vi "Auto Shooter Mode.vi"(0 "Shooter Command":T1, 9 "Ball Loaded?":bool) -> (8 "Secure Ball?":bool, 10 "Angle In Range?":bool, 11 "RPM Ready?":bool, 12 "Vision Target Aligned?":bool, 13 "Intake High Angle Allowed?":bool, 14 "State":T5, 15 "Shooter Ready?":bool, 16 "Left Output":dbl, 17 "Right Output":dbl, 18 "Angle Motor Output":dbl, 19 "Trigger Output":dbl)   [LabVIEW 2015]
uses:
  Common Code/Shooter State.ctl
  Common Code/Shooter Command Cluster.ctl
  Common Code/Shooter Commands.ctl
  Common Code/Shoot Modes Enum.ctl
  Common Code/Shot Type.ctl
  Common Code/Change Detect Int.vi
  Common Code/Change Detect Boolean.vi
  Robot Global Data.vi
panel:
  out "Ball Loaded? 2":bool
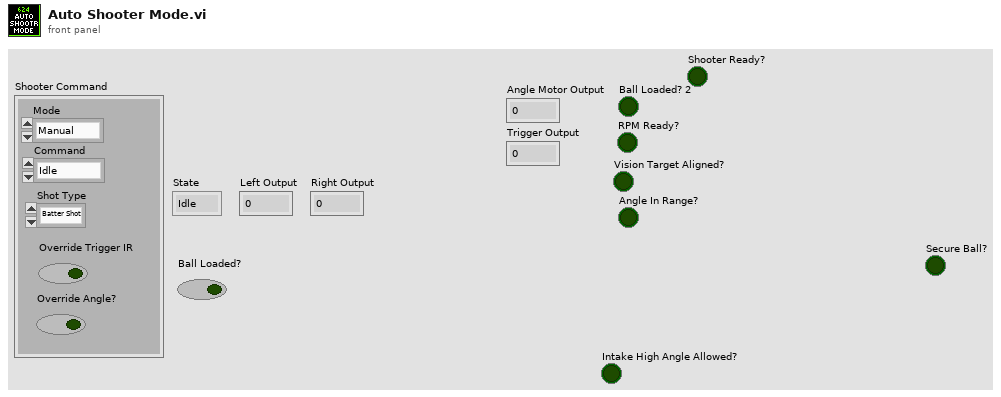
[diagram p1: front panel]
types:
  T1 = typedef "Shooter Command Cluster.ctl" = cluster{"Command":T2, "Mode":T3, "Shot Type":T4, "Override Trigger IR":bool, "Override Angle?":bool}
  T2 = typedef "Shooter Commands.ctl" = enum16{"Idle", "Prime Shooter", "Shoot"}
  T3 = typedef "Shoot Modes Enum.ctl" = enum16{"Manual", "Safe", "Auto"}
  T4 = typedef "Shot Type.ctl" = enum16{"Batter Shot", "Corner Shot", "Curve Shot", "Vision Shot", "Deep Middle Shot"}
  T5 = typedef "Shooter State.ctl" = enum16{"Idle", "Warmup", "Shooter Ready", "Shoot"}
  T6 = typedef "Intake Status Cluster.ctl" = cluster{"Roller Power":dbl, "Angle Power":dbl, "Intake Mode":T7, "Intake States":T8, "Rollers Active?":bool, "Current Height":dbl, "Target Height":dbl, "Encoder Raw Position":dbl, "Forward Tripped?":bool, "Backward Tripped?":bool, "Override IR?":bool}
  T7 = typedef "Intake Mode.ctl" = enum16{"Safe", "Auto", "Manual"}
  T8 = typedef "Intake States.ctl" = enum16{"Idle", "Set roller speed", "Move to angle"}
  T9 = typedef "Drivetrain Status Cluster.ctl" = cluster{"Modes":T10, "Y (Throttle)":dbl, "X (Steer)":dbl, "Gyro In Range?":bool, "Distance Drive Finished?":bool, "Stop Eject Lockout":bool, "Dist Drive Status":T11, "Y Target":dbl, "Heading Target":dbl, "Vision Target Aligned?":bool, "Gear":dbl, "1st Gear Time":dbl, "2nd Gear Time":dbl, "1st Gear Shifts":dbl, "2nd Gear Shifts":dbl}
  T10 = typedef "Drivetrain Modes.ctl" = enum16{"Climb", "Manual", "Ball Vision Targeting", "Goal Vision Targeting", "PID Distance Drive", "Hybrid"}
  T11 = typedef "Dist Drive Status.ctl" = cluster{"Y In Range":bool, "X In Range":bool, "Gyro In Range":bool, "Y Dist":dbl, "X Dist":dbl, "Gyro":dbl}
  T12 = typedef "Dashboard Control Data.ctl" = cluster{"Shooter Presets":T13, "Encoder Control":T15, "Steer PID output":cluster{"output high":dbl, "output low":dbl}, " Steer PID gains":cluster{"proportional gain (Kc)":dbl, "integral time (Ti, min)":dbl, "derivative time (Td, min)":dbl}, "Drivetrain Settings":T16, "Vision Packet":T17, "Dashboard Drivetrain Command":T18, "Info/Command Cluster":T20, "Ball Vision Packet":T21, "Intake Presets":T23, "Intake Encoder Control":T25, "Climb Presets":T26, "Ultrasonic Limit":dbl, "Roll Limit":dbl, "Pitch Limit":dbl, "Goal Output Range":cluster{"output high":dbl, "output low":dbl}}
  T13 = typedef "Shooter Presets.ctl" = cluster{"Batter Shot":T14, "Deep Middle Shot":T14, "Manual Shot":T14, "Left Ticks Per Rotation":dbl, "Right Ticks Per Rotation":dbl, "Low Bar Shot":T14, "Shooter RPM Tolerance":dbl, "IIR Filter Power":dbl, "Trigger Power":dbl, "Fire from Load Delay":i32, "Angle Pot M":dbl, "Angle Pot B":dbl, "Shooter Length":dbl, "String Pot Dist":dbl, "Angle PID gains":cluster{"proportional gain (Kc)":dbl, "integral time (Ti, min)":dbl, "derivative time (Td, min)":dbl}, "Angle Motor Output":cluster{"output high":dbl, "output low":dbl}, "Shooter Angle Tolerance":dbl, "Vision Shoot x^2":dbl, "Vision Shoot x":dbl, "Dist from Axis Cam to Pivot":dbl, "High Goal Center Height":dbl, "Feed Forward Max Accel":dbl, "Feed Forward Kv":dbl, "Backwards Trigger":dbl, "Shot Finish Delay (ms)":dbl, "Angle Max Current":dbl, "Angle Current Trip Time":dbl, "Shooter Intake Angle":dbl, "Vision Shoot c":dbl, "Reset?":bool, "Servo Release Delay":dbl, "Servo Idle Angle":i32, "Servo Hold Angle":i32, "Angle Pot x^2":dbl, "Angle Pot x":dbl, "Angle Pot c":dbl, "Ignore Angle?":bool}
  T14 = typedef "Shot Presets.ctl" = cluster{"Left Wheel RPM":dbl, "Right Wheel RPM":dbl, "Angle":dbl}
  T15 = typedef "Encoder Control.ctl" = cluster{"Right Tick Constant":dbl, "Left Tick Constant":dbl, "Reset?":bool, "Y Dist":cluster{"PID gains":cluster{"proportional gain (Kc)":dbl, "integral time (Ti, min)":dbl, "derivative time (Td, min)":dbl}}, "Y Stop Thresh":dbl, "Y Stop Speed":dbl}
  T16 = typedef "Drivetrain Settings.ctl" = cluster{"Gyro Tolerance":dbl, "Throttle Ramp (ms)":dbl, "Angular rate compensation":bool, "Throttle to Rate Scale":dbl, "Rate compensation gain":dbl, "Kv":dbl, "Ka":dbl, "Feed Forward P":dbl, "Feed Forward D":dbl, "Goal Vision PID gains":cluster{"proportional gain (Kc)":dbl, "integral time (Ti, min)":dbl, "derivative time (Td, min)":dbl}, "Goal Detection Window":dbl}
  T17 = typedef "Goal Vision Packet.ctl" = cluster{"Distance":dbl, "Center X":dbl, "Center Y":dbl, "Found Target?":bool}
  T18 = typedef "Dashboard Drivetrain Command.ctl" = cluster{"Drivetrain Vision":T19}
  T19 = typedef "Drivetrain Vision.ctl" = cluster{"Goal Window":dbl, "Ball Window":dbl}
  T20 = typedef "Ball Tracking Command Cluster.ctl" = cluster{"Distance to Ball":dbl, "Desired Angle":dbl, "Command":enum16{"Turn to Ball", "Turn to Angle", "Get Distance"}, "Pixels from Center":dbl}
  T21 = typedef "Ball Vision Packet.ctl" = cluster{"Ball Detected?":bool, "Distance to Ball":dbl, "Desired Angle":dbl, "Pixels from Center":dbl, "Tracking mode":T22}
  T22 = typedef "Tracking Mode.ctl" = enum16{"Turn to Ball", "Turn to Angle"}
  T23 = typedef "Intake Presets.ctl" = cluster{"Intake Speed":dbl, "Outake Speed":dbl, "Low Height":dbl, "Half Height":dbl, "Full Height":dbl, "Angle Speed":dbl, "Fast Angle":dbl, "Encoder Scale":dbl, "Load Height":dbl, "Output Range":T24, "Rotation Power Max/Min":dbl, "MaxCurrent":dbl, "Intake Trip Time":dbl, "Idle Height":dbl, "Max Height":dbl, "Reset Encoders?":bool, "PID gains":cluster{"proportional gain (Kc)":dbl, "integral time (Ti, min)":dbl, "derivative time (Td, min)":dbl}}
  T24 = typedef "Drivetrain Output Range.ctl" = cluster{"output high":dbl, "output low":dbl}
  T25 = typedef "IntakeEcoderControl.ctl" = cluster{"Arm Tick Constant":dbl, "Reset?":bool, "Y Dist":cluster{"PID gains":cluster{"proportional gain (Kc)":dbl, "integral time (Ti, min)":dbl, "derivative time (Td, min)":dbl}}, "Y Stop Thresh":dbl, "Y Stop Speed":dbl}
  T26 = typedef "Climb Presets.ctl" = cluster{"Pull Power":dbl, "Unpin Power":dbl, "Time to Hold":dbl}
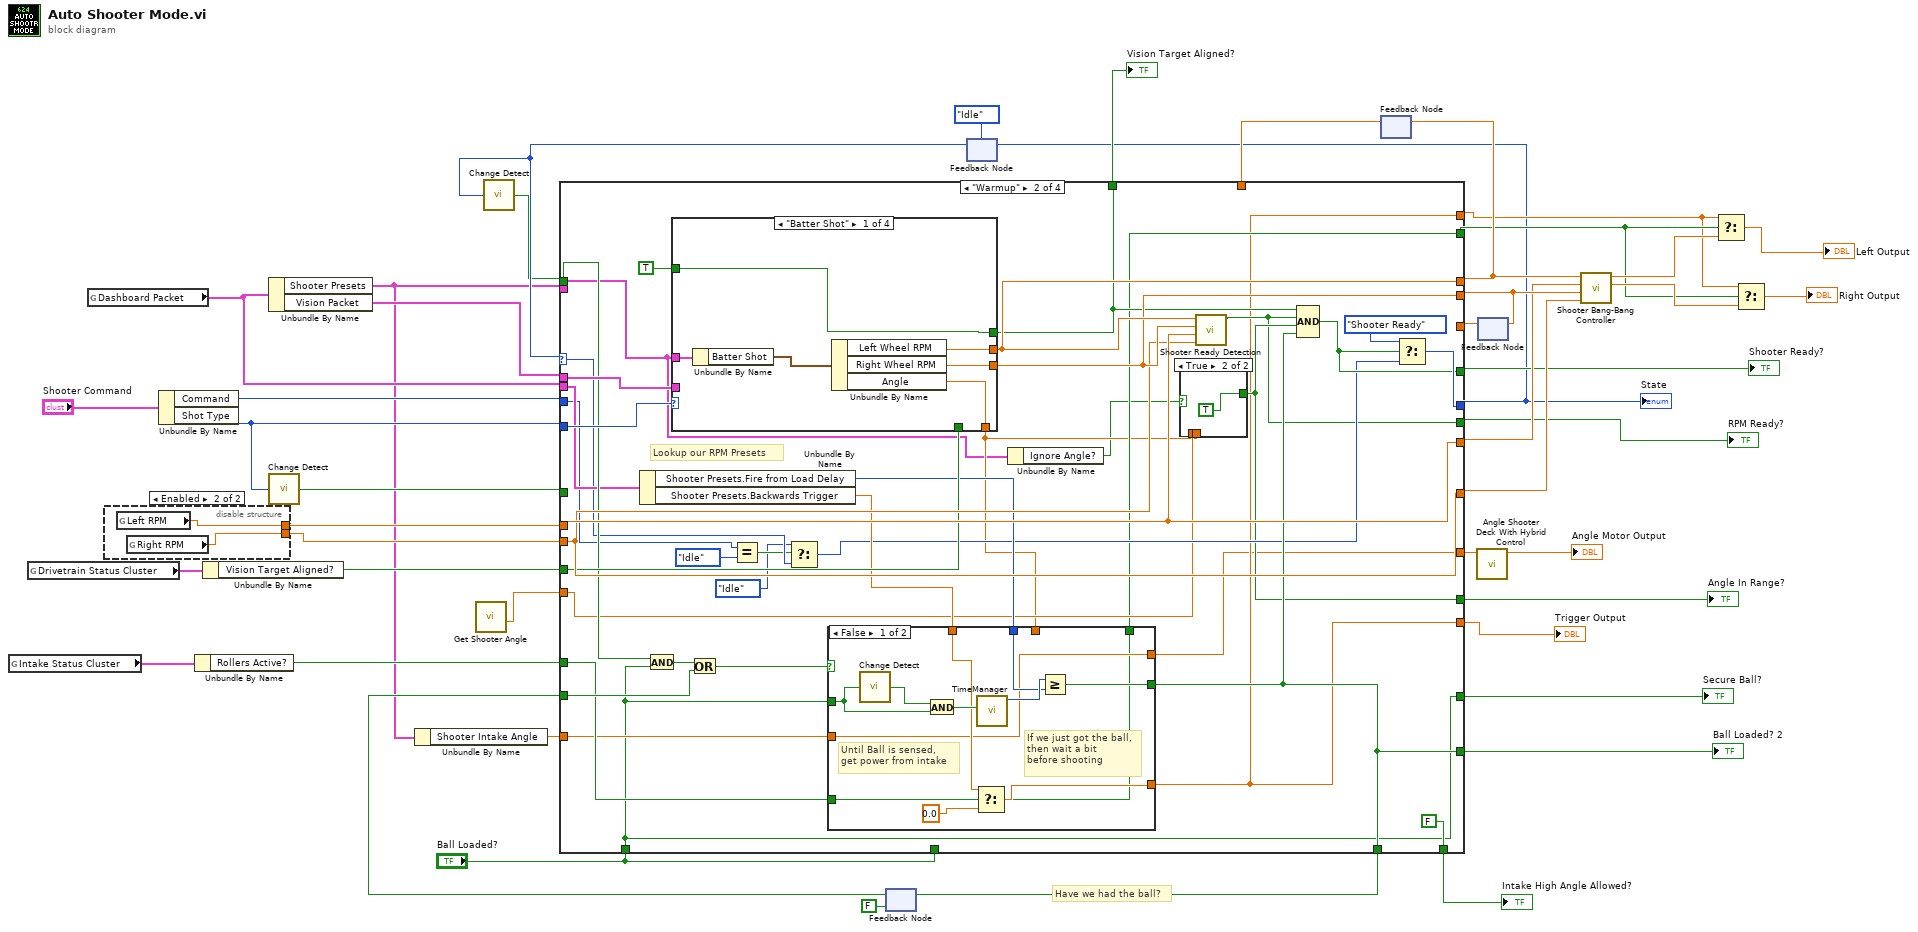
[diagram p0: block diagram]
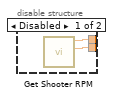
[diagram p2: hidden frame]
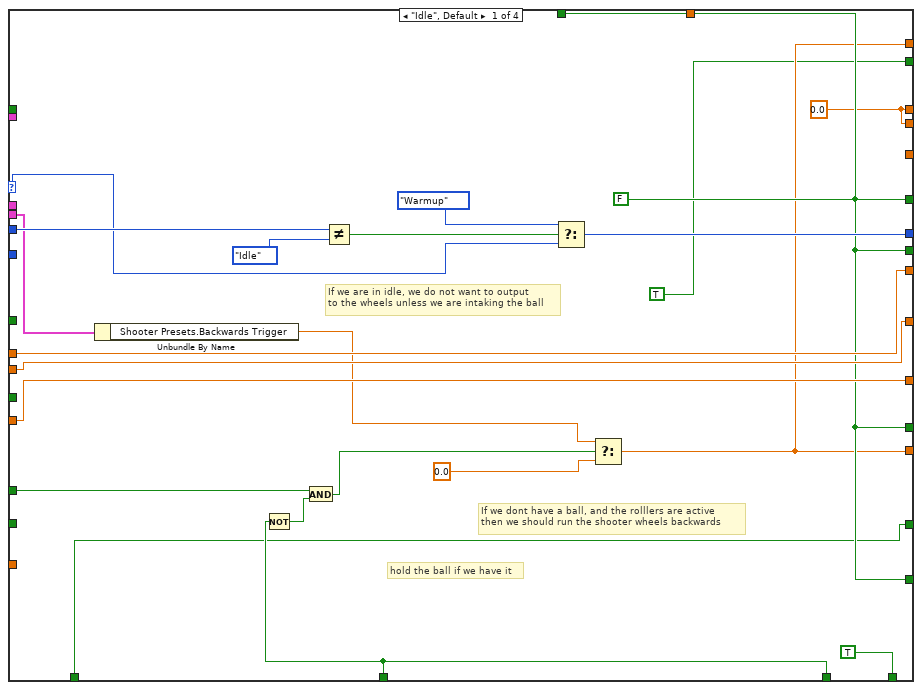
[diagram p3: hidden frame]
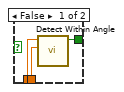
[diagram p4: hidden frame]
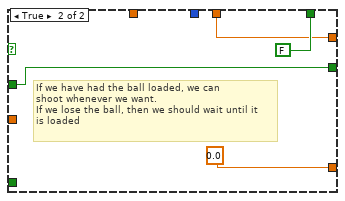
[diagram p5: hidden frame]
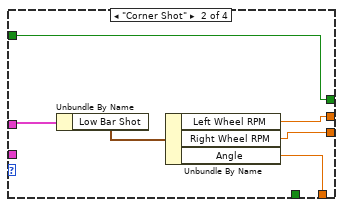
[diagram p6: hidden frame]
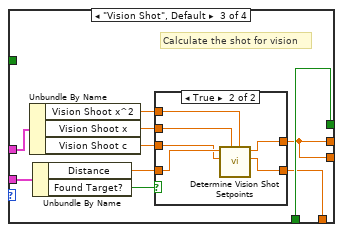
[diagram p7: hidden frame]
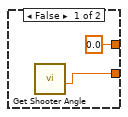
[diagram p8: hidden frame]
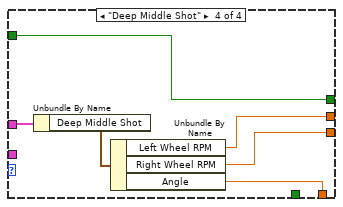
[diagram p9: hidden frame]
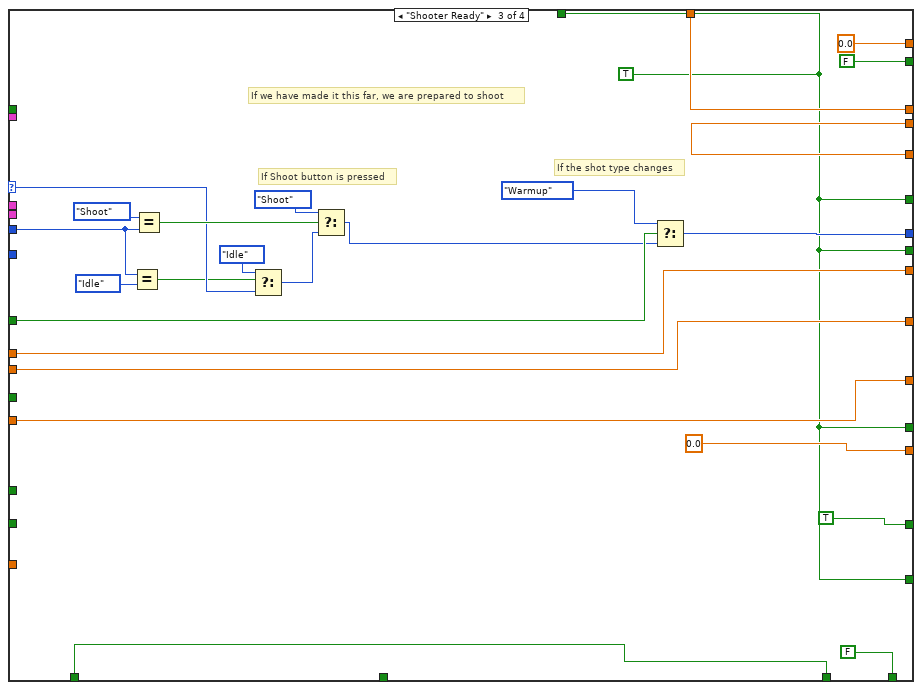
[diagram p10: hidden frame]
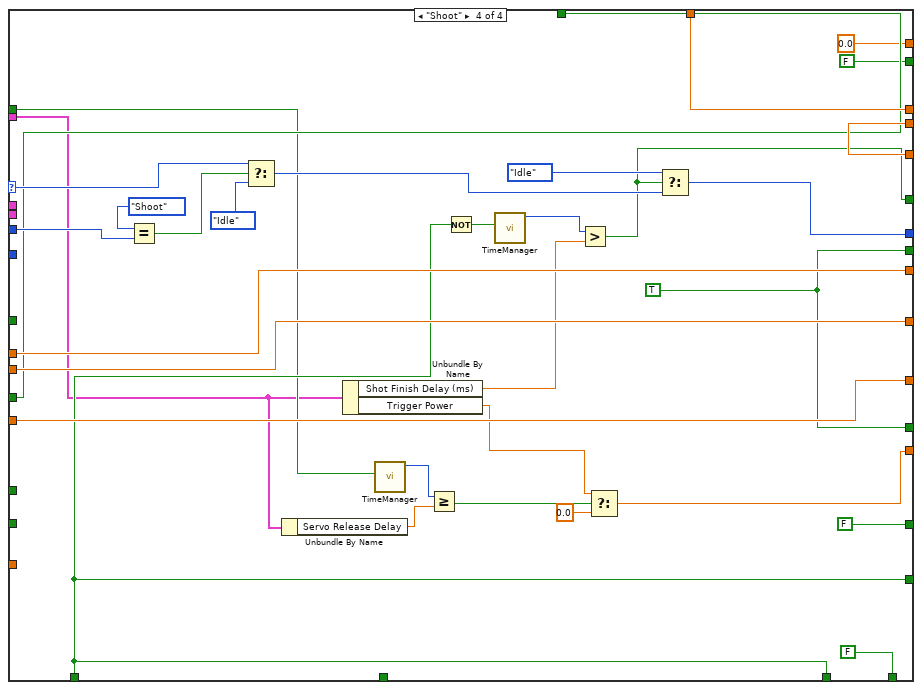
[diagram p11: hidden frame]
diagram:
  # "Have we had the ball?"
  n1 = global read "Robot Global Data.vi" "Intake Status Cluster"() -> (w5:T6)
  n2 = global read "Robot Global Data.vi" "Drivetrain Status Cluster"() -> (w32:T9)
  n3 = global read "Robot Global Data.vi" "Dashboard Packet"() -> (w7:T12)
  n4 = disable-structure shown="Enabled" {
    disable-tunnel: [w47 w48] -> w36
    disable-tunnel: [w46 w49] -> w35
    frame Disabled {
      n5 = call "Get Shooter RPM.vi"() -> ("Right RPM"=w46:dbl, "Left RPM"=w47:dbl)  [unwired: 9 in, 1 out]
    }
    frame Enabled {
      n6 = global read "Robot Global Data.vi" "Left RPM"() -> (w48:dbl)
      n7 = global read "Robot Global Data.vi" "Right RPM"() -> (w49:dbl)
    }
  }
  n8 = Unbundle By Name("Shooter Command") -> ("Command"=w44:T2, "Shot Type"=w42:T4)
  n9 = Unbundle By Name(w5) -> ("Rollers Active?"=w30:bool)
  n10 = Unbundle By Name(w32) -> ("Vision Target Aligned?"=w31:bool)
  n11 = Unbundle By Name(w7) -> ("Shooter Presets"=w6:T13, "Vision Packet"=w20:T17)
  n12 = call-poly "Change Detect.vi"("In"=w42) -> ("Changed?"=w41:bool)
  n13 = Unbundle By Name(w6) -> ("Shooter Intake Angle"=w4:dbl)
  n14 = call "Get Shooter Angle.vi"() -> ("Current Angle"=w8:dbl)  [unwired: 11 in]
  n15 = feedback #1(FALSE ("Ball Loaded?")) -> (w26:bool)
  n16 = feedback #2(Shooter_State."Idle") -> (w24:T5)
  n17 = call-poly "Change Detect.vi"("In"=w24) -> ("Changed?"=w23:bool)
  n18 = feedback #3() -> (w39:dbl)  [unwired: 1 in]
  n19 = feedback #4() -> (w37:dbl)  [unwired: 1 in]
  n20 = case shown="\"Warmup\"" w24 {
    selector: w24 -> [w64 w89 w174 w219]
    tunnel: w44 -> [w67 w86 w182 w222]
    tunnel: [w69 w106 w187 w212] -> w1
    tunnel: w6 -> [_ w73 _ w198]
    tunnel: w42 -> [_ w110 _ _]
    tunnel: [w55 w108 w185 w217] -> w38
    tunnel: [w55 w109 w186 w218] -> w40
    tunnel: w41 -> [_ _ w189 _]
    tunnel: w39 -> [_ _ w186 w218]
    tunnel: w37 -> [_ _ w185 w217]
    tunnel: w36 -> [w66 w105 w184 w216]
    tunnel: w35 -> [w65 w104 w183 w215]
    tunnel: [w66 w105 w184 w216] -> w34
    tunnel: [w65 w104 w183 w215] -> w33
    tunnel: w31 -> [_ w100 _ w208]
    tunnel: "Ball Loaded?" -> [w61 _ _ _]
    tunnel: w20 -> [_ w103 _ _]
    tunnel: [w62 w77 w176 w211] -> w21
    tunnel: w30 -> [w60 w93 _ _]
    tunnel: [w53 w79 0.0 ("f") w192] -> w29
    tunnel: "Ball Loaded?" -> [w50 w74 w181 w202]
    tunnel: w7 -> [w58 w90 _ _]
    tunnel: [w61 w98 w181 w202] -> w27
    tunnel: w26 -> [_ w95 _ _]
    tunnel: w23 -> [_ w94 _ w199]
    tunnel: w8 -> [w62 w82 w176 w211]
    tunnel: [w57 w102 w170 w201] -> w19
    tunnel: [w57 w83 w170 w209] -> w18
    tunnel: [w57 w81 w170 w209] -> w17
    tunnel: [w57 w98 w170 w202] -> w16
    tunnel: [w57 w101 w170 w208] -> w15
    tunnel: [TRUE w80 FALSE FALSE] -> w12
    tunnel: [w53 w79 0.0 ("f") 0.0 ("f")] -> w11
    tunnel: w4 -> [_ w76 _ _]
    tunnel: [TRUE ("Intake High Angle Allowed?") FALSE ("Intake High Angle Allowed?") FALSE ("Intake High Angle Allowed?") FALSE ("Intake High Angle Allowed?")] -> w3
    tunnel: [w50 w74 TRUE ("Intake High Angle Allowed?") FALSE ("Intake High Angle Allowed?")] -> w2
    frame "Idle", Default {
      w55 = 0.0 ("Left Wheel RPM")
      w57 = FALSE ("Shooter Ready?")
      # "hold the ball if we have it"
      # "If we dont have a ball, and the rolllers are active\nthen we should run the shooter wheels backwards"
      # "If we are in idle, we do not want to output\nto the wheels unless we are intaking the ball"
      n21 = Unbundle By Name(w58) -> ("Shooter Presets.Backwards Trigger"=w56:dbl)
      n22 = Not(x=w61) -> (.not. x?=w59:bool)
      n23 = And(x=w60, y=w59) -> (x .and. y?=w54:bool)
      n24 = Not Equal?(x=w67, y=Shooter_Commands."Idle" ("Command")) -> (x != y?=w70:bool)
      n25 = Select(t=Shooter_State."Warmup", s=w70, f=w64) -> (s? t:f=w69:T5)
      n26 = Select(t=w56, s=w54, f=0.0) -> (s? t:f=w53:dbl)
    }
    frame "Warmup" {
      # "Lookup our RPM Presets"
      n27 = Unbundle By Name(w90) -> ("Shooter Presets.Fire from Load Delay"=w92:i32, "Shooter Presets.Backwards Trigger"=w91:dbl)
      n28 = And(x=w94, y=w74) -> (x .and. y?=w96:bool)
      n29 = case shown="\"Batter Shot\"" w110 {
        tunnel: w73 -> [w135 w141 w150 w165]
        tunnel: [w133 w137 w145 w163] -> w109
        tunnel: [w132 w138 w145 w162] -> w108
        tunnel: w103 -> [_ _ w147 _]
        tunnel: [w131 w136 w151 w161] -> w101
        tunnel: w100 -> [_ _ w151 _]
        tunnel: TRUE -> [w131 w136 _ w161]
        tunnel: [w130 w139 w146 w160] -> w78
        frame "Batter Shot" {
          n30 = Unbundle By Name(w135) -> ("Batter Shot"=w134:T14)
          n31 = Unbundle By Name(w134) -> ("Left Wheel RPM"=w133:dbl, "Right Wheel RPM"=w132:dbl, "Angle"=w130:dbl)
        }
        frame "Corner Shot" {
          n32 = Unbundle By Name(w141) -> ("Low Bar Shot"=w140:T14)
          n33 = Unbundle By Name(w140) -> ("Left Wheel RPM"=w137:dbl, "Right Wheel RPM"=w138:dbl, "Angle"=w139:dbl)
        }
        frame "Vision Shot", Default {
          # "Calculate the shot for vision"
          n34 = Unbundle By Name(w150) -> ("Vision Shoot x^2"=w143:dbl, "Vision Shoot x"=w144:dbl, "Vision Shoot c"=w142:dbl)
          n35 = Unbundle By Name(w147) -> ("Distance"=w149:dbl, "Found Target?"=w148:bool)
          n36 = case shown="True" w148 {
            tunnel: w149 -> [_ w159]
            tunnel: [w152 w158] -> w146
            tunnel: [0.0 ("Power") w157] -> w145
            tunnel: w144 -> [_ w156]
            tunnel: w143 -> [_ w155]
            tunnel: w142 -> [_ w154]
            frame False {
              n37 = call "Get Shooter Angle.vi"() -> ("Current Angle"=w152:dbl)  [unwired: 11 in]
            }
            frame True {
              n38 = call "Determine Vision Shot Setpoints.vi"("x^2"=w155, "x"=w156, "c"=w154, "Distance from Target"=w159) -> ("Angle"=w158:dbl, "RPM Power"=w157:dbl)  [unwired: 6 in]
            }
          }
        }
        frame "Deep Middle Shot" {
          n39 = Unbundle By Name(w165) -> ("Deep Middle Shot"=w164:T14)
          n40 = Unbundle By Name(w164) -> ("Left Wheel RPM"=w163:dbl, "Right Wheel RPM"=w162:dbl, "Angle"=w160:dbl)
        }
      }
      n41 = Or(x=w96, y=w95) -> (x .or. y?=w97:bool)
      n42 = Equal?(x=w86, y=Shooter_Commands."Idle") -> (x = y?=w87:bool)
      n43 = Select(t=Shooter_State."Idle", s=w87, f=w89) -> (s? t:f=w88:T5)
      n44 = case shown="False" w97 {
        tunnel: w92 -> [w122 _]
        tunnel: w74 -> [w121 w129]
        tunnel: [w120 w129] -> w98
        tunnel: [w118 0.0 ("f")] -> w79
        tunnel: w93 -> [w115 _]
        tunnel: w91 -> [w117 _]
        tunnel: [w115 FALSE] -> w80
        tunnel: w78 -> [_ w126]
        tunnel: [w116 w126] -> w77
        tunnel: w76 -> [w116 _]
        frame False {
          # "Until Ball is sensed,\nget power from intake"
          # "If we just got the ball,\nthen wait a bit\nbefore shooting"
          n45 = call-poly "Change Detect.vi"("In"=w121) -> ("Changed?"=w125:bool)
          n46 = And(x=w125, y=w121) -> (x .and. y?=w124:bool)
          n47 = Select(t=w117, s=w115, f=0.0 ("t")) -> (s? t:f=w118:dbl)
          n48 = call "TimeManager.vi"("Reset?"=w124) -> ("Time Since Reset"=w123:u32)  [unwired: 9 in, 1 out]
          n49 = Greater Or Equal?(x=w123, y=w122) -> (x >= y?=w120:bool)
        }
        frame True {
          # "If we have had the ball loaded, we can\nshoot whenever we want.\nIf we lose the ball, then we should wait until it\nis loaded"
        }
      }
      n50 = Unbundle By Name(w73) -> ("Ignore Angle?"=w72:bool)
      n51 = case shown="True" w72 {
        tunnel: [w113 TRUE ("In Range?")] -> w83
        tunnel: w82 -> [w112 _]
        tunnel: w78 -> [w111 _]
        frame False {
          n52 = call "Detect Within Angle.vi"("Angle Target"=w111, "Current Angle"=w112) -> ("In Range?"=w113:bool)  [unwired: 9 in]
        }
        frame True {
        }
      }
      n53 = call "Shooter Ready Detection.vi"("Right RPM"=w104, "Left RPM"=w105, "Right RPM Target"=w108, "Left RPM Target"=w109) -> ("Shooter Ready?"=w81:bool)  [unwired: 7 in]
      n54 = Compound Arithmetic op=AND(w101, w81, w83, w98) -> (w102:bool)
      n55 = Select(t=Shooter_State."Shooter Ready", s=w102, f=w88) -> (s? t:f=w106:T5)
    }
    frame "Shooter Ready" {
      w170 = TRUE ("Vision Target Aligned?")
      # "If the shot type changes"
      # "If Shoot button is pressed"
      # "If we have made it this far, we are prepared to shoot"
      n56 = Equal?(x=w182, y=Shooter_Commands."Idle") -> (x = y?=w173:bool)
      n57 = Equal?(x=Shooter_Commands."Shoot", y=w182) -> (x = y?=w180:bool)
      n58 = Select(t=Shooter_State."Idle", s=w173, f=w174) -> (s? t:f=w175:T5)
      n59 = Select(t=Shooter_State."Shoot", s=w180, f=w175) -> (s? t:f=w178:T5)
      n60 = Select(t=Shooter_State."Warmup", s=w189, f=w178) -> (s? t:f=w187:T5)
    }
    frame "Shoot" {
      w209 = TRUE ("Vision Target Aligned?")
      n61 = Equal?(x=Shooter_Commands."Shoot", y=w222) -> (x = y?=w220:bool)
      n62 = Select(t=w219, s=w220, f=Shooter_State."Idle") -> (s? t:f=w213:T5)
      n63 = Unbundle By Name(w198) -> ("Servo Release Delay"=w197:dbl)
      n64 = Unbundle By Name(w198) -> ("Shot Finish Delay (ms)"=w204:dbl, "Trigger Power"=w194:dbl)
      n65 = call "TimeManager.vi"("Reset?"=w199) -> ("Time Since Reset"=w196:u32)  [unwired: 9 in, 1 out]
      n66 = Greater Or Equal?(x=w196, y=w197) -> (x >= y?=w195:bool)
      n67 = Not(x=w202) -> (.not. x?=w205:bool)
      n68 = call "TimeManager.vi"("Reset?"=w205) -> ("Time Since Reset"=w203:u32)  [unwired: 9 in, 1 out]
      n69 = Greater?(x=w203, y=w204) -> (0:w201:bool)
      n70 = Select(t=w194, s=w195, f=0.0) -> (s? t:f=w192:dbl)
      n71 = Select(t=Shooter_State."Idle" ("f"), s=w201, f=w213) -> (s? t:f=w212:T5)
    }
  }
  "State" <- w1
  "Trigger Output" <- w29
  "Ball Loaded? 2" <- w16
  "Shooter Ready?" <- w19
  "RPM Ready?" <- w17
  "Angle In Range?" <- w18
  "Vision Target Aligned?" <- w15
  "Intake High Angle Allowed?" <- w3
  "Secure Ball?" <- w2
  n72 = feedback-in #1(w27) -> ()
  n73 = feedback-in #2(w1) -> ()
  n74 = feedback-in #3(w40) -> ()
  n75 = call "Angle Shooter Deck With Hybrid Control.vi"("Target Angle"=w21) -> ("Angle Motor Power Out"=→"Angle Motor Output":dbl)  [unwired: 10 in]
  n76 = feedback-in #4(w38) -> ()
  n77 = call "Shooter Bang-Bang Controller.vi"("Right Current RPM"=w33, "Right Target RPM"=w38, "Left Current RPM"=w34, "Left Target RPM"=w40) -> ("Right Output Power"=w13:dbl, "Left Output Power"=w14:dbl)  [unwired: 6 in]
  n78 = Select(t=w11, s=w12, f=w14) -> (s? t:f=→"Left Output":dbl)
  n79 = Select(t=w11, s=w12, f=w13) -> (s? t:f=→"Right Output":dbl)
